vi "Find Error and Warning.vi"(8 "error in (no error)":errorcluster, 11 "error code":i32) -> (0 "error out":errorcluster)   [LabVIEW 2017, in "HD44780 Common.lvlib"]
uses:
  HD44780 Common.lvlib
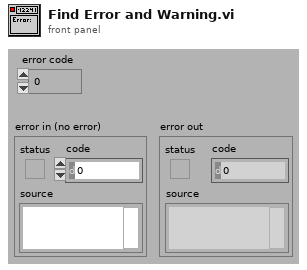
[diagram p1: front panel]
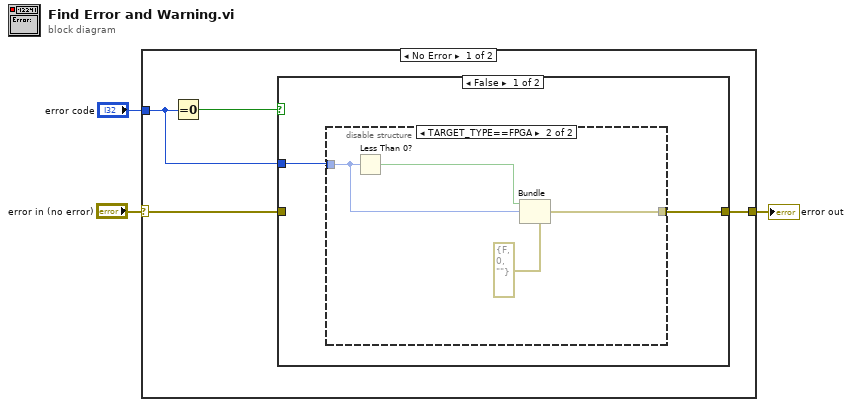
[diagram p0: block diagram]
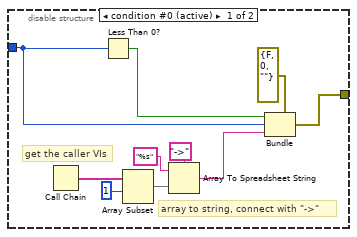
[diagram p2: hidden frame]
diagram:
  n1 = case shown="No Error" "error in (no error)" {
    selector: "error in (no error)" -> [w4 w25]
    tunnel: "error code" -> [w6 _]
    tunnel: [w7 w25] -> w2
    frame No Error {
      n2 = Equal To 0?(x=w6) -> (x = 0?=w5:bool)
      n3 = case shown="False" w5 {
        tunnel: [w9 w24] -> w7
        tunnel: w6 -> [w8 _]
        tunnel: w4 -> [_ w24]
        frame False {
          n4 = disable-structure shown="TARGET_TYPE==FPGA" {
            disable-tunnel: [w12 w22] -> w9
            disable-tunnel: w8 -> [w10 w20]
            frame condition #0 (active) {
              # "array to string, connect with \"->\""
              # "get the caller VIs"
              n5 = Call Chain() -> (call chain=w17:string[])
              n6 = Less Than 0?(x=w10) -> (x < 0?=w11:bool)
              n7 = Array Subset(array=w17, index=1 ("Array Index")) -> (w16:string[])  [unwired: 1 in]
              n8 = Array To Spreadsheet String(delimiter (Tab)="->", array=w16, 3:"%s" ("format string")) -> (spreadsheet string=w13:string)
              n9 = Bundle(cluster=errorcluster {"status"=FALSE, "code"=0, "source"=""} ("error in (no error)"), "status"=w11, "code"=w10, "source"=w13) -> (w12:errorcluster)
            }
            frame condition #1 {
              n10 = Less Than 0?(x=w20) -> (x < 0?=w21:bool)
              n11 = Bundle(cluster=errorcluster {"status"=FALSE, "code"=0, "source"=""} ("error in (no error)"), "status"=w21, "code"=w20) -> (w22:errorcluster)  [unwired: 1 in]
            }
          }
        }
        frame True {
        }
      }
    }
    frame Error {
    }
  }
  "error out" <- w2
